vi "Init.vi"(8 "error in (no error)":errorcluster, 10 "Address":string, 11 "ArduinoTranslationStage in":refnum<class "ArduinoTranslationStage.lvclass">) -> (0 "error out":errorcluster, 3 "ArduinoTranslationStage out":refnum<class "ArduinoTranslationStage.lvclass">)   [LabVIEW 2023, in "ArduinoTranslationStage.lvlib" / "ArduinoTranslationStage.lvclass"]
uses:
  ArduinoTranslationStage.lvclass
  ArduinoTranslationStage.lvclass/ArduinoTranslationStage.ctl
  <vilib>/Instr/_visa.llb/Select Event Type.ctl
  Cameras_LV/InitDeinitComm Messages/InitDone Msg/InitDone Msg.lvclass
  <vilib>/ActorFramework/Actor/Actor.lvclass
  Applications/National Instruments/LabVIEW 2023 64-bit/vi.lib/ActorFramework/Actor/Actor.lvclass
  Users/alexandrosspiliotis/Documents/TranslationStage/ArduinoTranslationStageActor/ArduinoTranslationStage Actor/ArduinoTranslationStage.lvclass
  Users/alexandrosspiliotis/Documents/Cameras_LV/InitDeinit/InitDeinit.lvclass
  Users/alexandrosspiliotis/Documents/TranslationStage/StepperMotorController/StepperMotorController.lvclass
  Users/alexandrosspiliotis/Documents/TranslationStage/TranslationStages/TranslationStagesInterface.lvclass
panel:
  in  "Address":T1
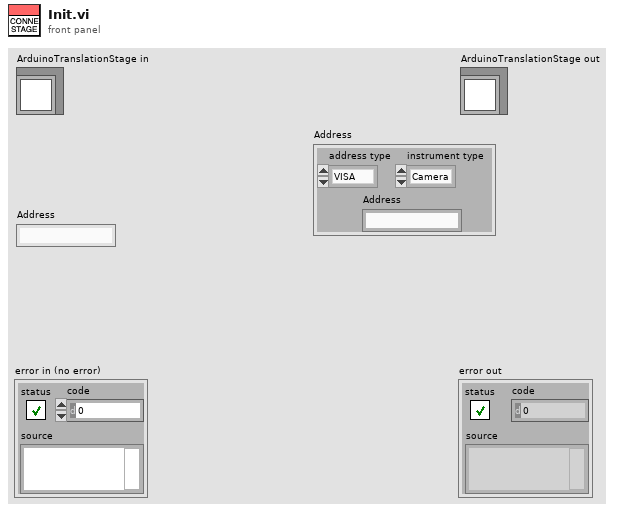
[diagram p1: front panel]
types:
  T1 = cluster{"address type":enum16{"VISA", "Index"}, "Address":string, "instrument type":enum16{"Camera", "Stepper"}}
  T2 = typedef "Select Event Type.ctl" = u32
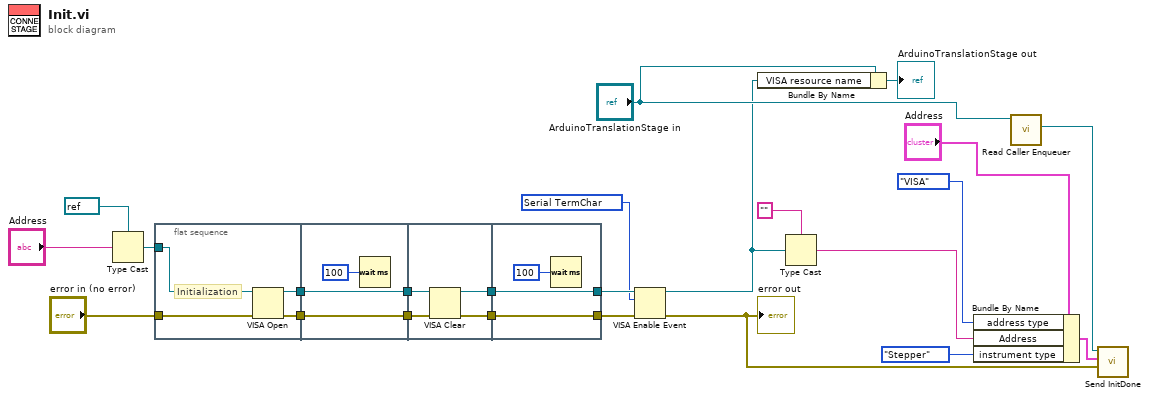
[diagram p0: block diagram]
diagram:
  w16 = T2 1073684516 items=["Service Request"=1073684491, "Trigger"=3221168138, "Clear"=1073684493, "VXI Signal"=1073684512, "VXI/VME Interrupt"=3221168161, "VXI/VME Sysfail"=1073684509, "VXI/VME Sysreset"=1073684510, "GPIB CIC"=1073684498, "GPIB Talk"=1073684499, "GPIB Listen"=1073684500, "PXI Interrupt"=1073684514, "Serial Break"=1073684515, "Serial TermChar"=1073684516, "Serial CTS"=1073684521, "Serial DSR"=1073684522, "Serial DCD"=1073684524, "Serial RI"=1073684526, "Serial Character"=1073684533, "USB Interrupt"=1073684535, "All Enabled"=1073709055] ("Event Type")
  n1 = Type Cast(type=refnum<visa-resource-name> refnum ("VISA resource name"), x="Address") -> (*(type *) &x=w13:refnum<visa-resource-name>)
  n2 = flat-sequence {
    tunnel: [w28] -> w24
    tunnel: [w27] -> w23
    tunnel: w13 -> [w26]
    tunnel: "error in (no error)" -> [w25]
    tunnel: [w30] -> w22
    tunnel: w24 -> [w30]
    tunnel: [w29] -> w21
    tunnel: w23 -> [w29]
    tunnel: [w33] -> w20
    tunnel: [w32] -> w19
    tunnel: w22 -> [w35]
    tunnel: w21 -> [w34]
    tunnel: [w37] -> w17
    tunnel: [w38] -> w18
    tunnel: w20 -> [w38]
    tunnel: w19 -> [w37]
    frame #0 {
      # "Initialization"
      n3 = VISA Open(error in (no error)=w25, VISA resource name=w26) -> (VISA resource name=w27:refnum<visa-resource-name>, error out=w28:errorcluster)  [unwired: 3 in]
    }
    frame #1 {
      n4 = Wait (ms)(milliseconds to wait=u32 100) -> ()  [unwired: 1 out]
    }
    frame #2 {
      n5 = VISA Clear(VISA resource name=w34, error in (no error)=w35) -> (VISA resource name out=w32:refnum<visa-resource-name>, error out=w33:errorcluster)
    }
    frame #3 {
      n6 = Wait (ms)(milliseconds to wait=u32 100) -> ()  [unwired: 1 out]
    }
  }
  n7 = VISA Enable Event(8:w18, 10:w16, 11:w17) -> (0:w4:errorcluster, 3:w8:refnum<visa-resource-name>)  [unwired: 1 in]
  "error out" <- w4
  n8 = Bundle By Name(cluster="ArduinoTranslationStage in", "VISA resource name"=w8) -> (→"ArduinoTranslationStage out":refnum<class "ArduinoTranslationStage.lvclass">)
  n9 = Type Cast(type="", x=w8) -> (*(type *) &x=w3:string)
  n10 = Bundle By Name(cluster="Address", "address type"=enum16{"VISA", "Index"}."VISA", "Address"=w3, "instrument type"=enum16{"Camera", "Stepper"}."Stepper" ("Stepper.instrument type")) -> (w5:T1)
  n11 = call <vilib>:"Read Caller Enqueuer.vi"("Actor"="ArduinoTranslationStage in") -> ("Caller Enqueuer"=w10:refnum<class "Message Enqueuer.lvclass">)  [unwired: 10 in]
  n12 = call "Send InitDone.vi"("instr error"=w4, "Address"=w5, "Message Enqueuer"=w10) -> ()  [unwired: 7 in, 2 out]
